vi "TCP Send Response.vi"(8 "error in (no error)":errorcluster, 10 "Response":string, 11 "connection ID":T1) -> (0 "error out":errorcluster, 3 "connection ID(dup)":T1)   [LabVIEW 2020, in "CSM-TCP-Router.lvlib"]
uses:
  CSM-TCP-Router.lvlib
  <vilib>/addons/_JKI.lib/_JKI_lib_TCP_Server.llb/TCP Server Connection Session ID Cluster.ctl
  tcp-msg type.ctl
  <userlib>/_NEVSTOP/Communicable State Machine(CSM)/AdvanceAPI/CSM - Make String Arguments Safe.vi
  <userlib>/_NEVSTOP/Communicable State Machine(CSM)/AdvanceAPI/CSM - Keywords.vi
  <userlib>/_NEVSTOP/Communicable State Machine(CSM)/Communicable State Machine.lvlib
  <vilib>/addons/_JKI.lib/_JKI_lib_TCP_Server.llb/JKI TCP Server.lvclass
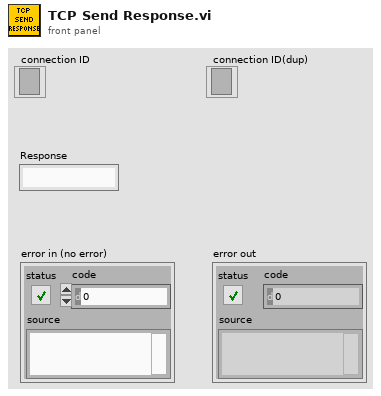
[diagram p1: front panel]
types:
  T1 = typedef "JKI TCP Server.lvclass/TCP Server Connection Session ID Cluster.ctl" = refnum<k5>
  T2 = typedef "CSM-TCP-Router.lvlib/tcp-msg type.ctl" = enum8{"info", "error", "cmd", "cmd-resp", "resp", "async-resp", "status", "interrupt"}
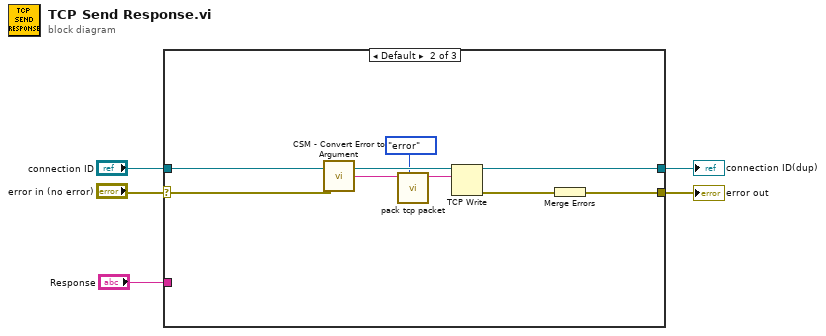
[diagram p0: block diagram]
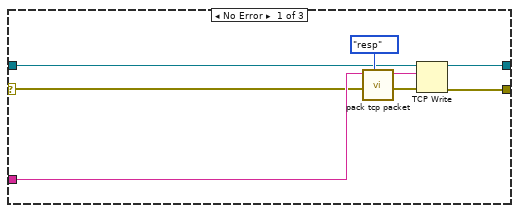
[diagram p2: hidden frame]
diagram:
  n1 = case shown="Default" "error in (no error)" {
    selector: "error in (no error)" -> [w6 w13 w21]
    tunnel: "connection ID" -> [w7 w20 w22]
    tunnel: [w9 w14 w21] -> w4
    tunnel: [w8 w17 w22] -> w5
    tunnel: "Response" -> [w10 _ _]
    frame No Error {
      n2 = call "pack tcp packet.vi"("tcp-message-type"=tcp-msg_type."resp", "String"=w10) -> ("TCP Pack"=w11:string)  [unwired: 9 in]
      n3 = TCP Write(connection ID=w7, data in=w11, error in (no error)=w6) -> (connection ID out=w8:T1, error out=w9:errorcluster)  [unwired: 1 in, 1 out]
    }
    frame Default {
      n4 = call <userlib>:"CSM - Convert Error to Argument.vi"("error"=w13) -> ("Argument"=w18:string)  [unwired: 4 in]
      n5 = call "pack tcp packet.vi"("tcp-message-type"=tcp-msg_type."error", "String"=w18) -> ("TCP Pack"=w16:string)  [unwired: 9 in]
      n6 = TCP Write(connection ID=w20, data in=w16) -> (connection ID out=w17:T1, error out=w19:errorcluster)  [unwired: 2 in, 1 out]
      n7 = Merge Errors(w19) -> (w14:errorcluster)
    }
    frame Error {
    }
  }
  "connection ID(dup)" <- w5
  "error out" <- w4
